vi "setUp.vi"(8 "error in (no error)":errorcluster, 11 "reference in":refnum<class "SMO_TestCase.lvclass">) -> (0 "error out":errorcluster, 3 "reference out":refnum<class "SMO_TestCase.lvclass">)   [LabVIEW 2013, in "SMO_TestCase.lvclass"]
doc: "setUp runs prior to the test method during test execution. Use this method to initialize any object data required by your tests."
uses:
  SMO_TestCase.lvclass
  Projects/JKI SMO Git/JKI-State-Machine-Objects/src/SMO/SMO.lvclass
  SMO_TestCase.lvclass/SMO_TestCase.ctl
  <vilib>/addons/_JKI Toolkits/VI Tester/TestCase.llb/TestCase.lvclass
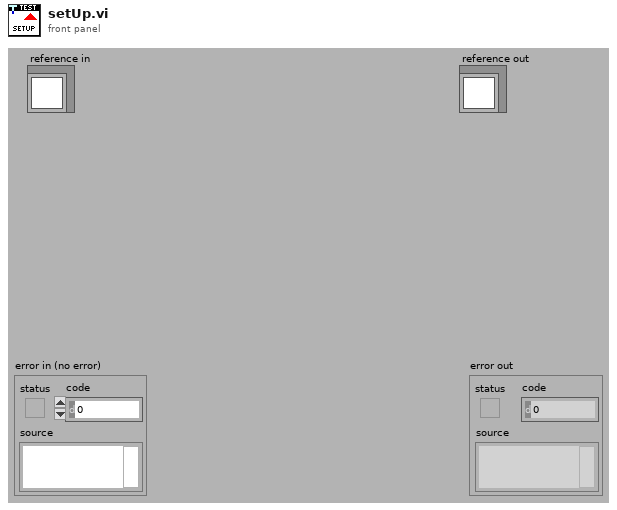
[diagram p1: front panel]
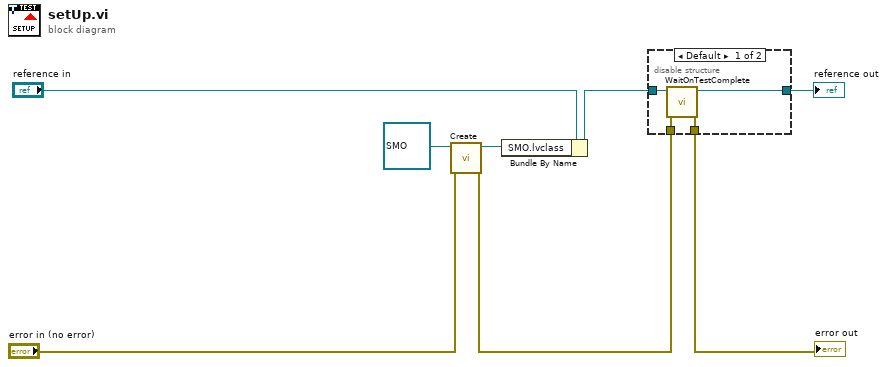
[diagram p0: block diagram]
diagram:
  n1 = call "Create.vi"("error in (no error)"="error in (no error)", "SMO"=refnum<class "SMO.lvclass"> refnum) -> ("error out"=w5:errorcluster, "SMO out"=w2:refnum<class "SMO.lvclass">)  [unwired: 8 in]
  n2 = Bundle By Name(cluster="reference in", "SMO.lvclass"=w2) -> (w3:refnum<class "SMO_TestCase.lvclass">)
  n3 = disable-structure shown="Default" {
    disable-tunnel: w5 -> [w12 w13]
    disable-tunnel: [w11 w13] -> w8
    disable-tunnel: [w10 w14] -> w7
    disable-tunnel: w3 -> [w9 w14]
    frame condition #0 (active) {
      n4 = call <vilib>:"WaitOnTestComplete.vi"("error in (no error)"=w12, "TestCase in"=w9) -> ("error out"=w11:errorcluster, "TestCase out"=w10:refnum<class "SMO_TestCase.lvclass">)  [unwired: 8 in]
    }
    frame condition #1 {
    }
  }
  "error out" <- w8
  "reference out" <- w7
